vi "Read Permissions.vi"(8 "Error In":errorcluster, 11 "File Info In":refnum<class "File Info.lvclass">) -> (0 "Error Out":errorcluster, 2 "Permissions":T1, 3 "File Info Out":refnum<class "File Info.lvclass">)   [LabVIEW 2021, in "Field_RnD_Services_LIBSSH2_Toolkit.lvlib" / "File Info.lvclass"]
doc: "Gets the POSIX-style filesystem permissions, or mode."
uses:
  220524-VNA RP FLAT.llb/File Info.lvclass
  220524-VNA RP FLAT.llb/Permissions.ctl
  Field_RnD_Services_LIBSSH2_Toolkit/Modes.ctl
  220524-VNA RP FLAT.llb/File Info.lvclass/File Info.ctl
  220524-VNA RP FLAT.llb/Field_RnD_Services_LIBSSH2_Toolkit.lvlib
  220524-VNA RP FLAT.llb/SSH.lvclass
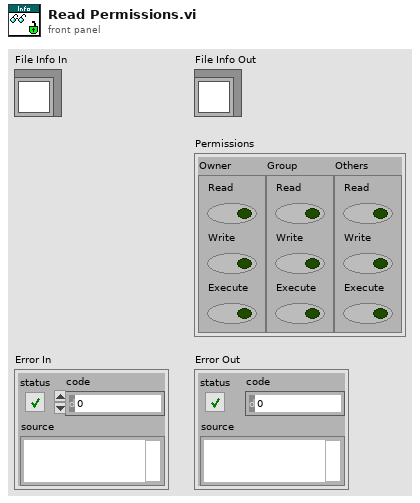
[diagram p1: front panel]
types:
  T1 = typedef "Field_RnD_Services_LIBSSH2_Toolkit.lvlib/Permissions.ctl" = cluster{"Owner":T2, "Group":T2, "Others":T2}
  T2 = typedef "Field_RnD_Services_LIBSSH2_Toolkit.lvlib/Modes.ctl" = cluster{"Read":bool, "Write":bool, "Execute":bool}
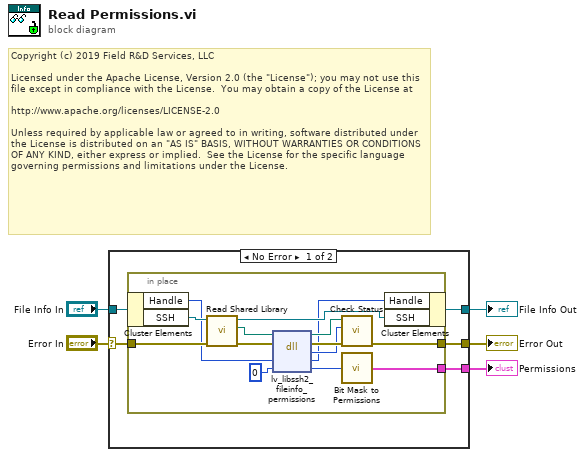
[diagram p0: block diagram]
diagram:
  # "Copyright (c) 2019 Field R&D Services, LLC\n\nLicensed under the Apache License, Version 2.0 (the \"License\"); you may not use this file except in compliance with the License.  You may obtain a copy of the License at\n\nhttp://www.apache.org/licenses/LICENSE-2.0\n\nUnless required by applicable law or agreed to in writing, software distributed under the License is distributed on an \"AS IS\" BASIS, WITHOUT WARRANTIES OR CONDITIONS OF ANY KIND, either express or implied.  See the License for the specific language governing permissions and limitations under the License."
  n1 = case shown="No Error" "Error In" {
    selector: "Error In" -> [w9 w26]
    tunnel: [w7 w26] -> w4
    tunnel: "File Info In" -> [w10 w25]
    tunnel: [w8 w25] -> w2
    tunnel: [w6 _] -> w1
    frame No Error {
      n2 = in-place {
        in-place-border: w9 -> [w17]
        in-place-border: [w14] -> w7
        in-place-border: [w11] -> w6
        n3 = in-place-cluster #1(w10) -> ("Handle"=w16:u64, "SSH"=w21:refnum<class "SSH.lvclass">)
        n4 = call "Read Shared Library.vi"("Error In"=w17, "SSH In"=w21) -> ("Error Out"=w18:errorcluster, "libssh2lv Shared Library"=w19:path, "SSH Out"=w20:refnum<class "SSH.lvclass">)  [unwired: 7 in]
        n5 = dll-call lib="lv-libssh2.*" fn="lv_libssh2_fileinfo_permissions"(path in=w19, error in=w18, "handle"=w16, "permissions"=u32 0 ("flags")) -> (path out=w23:path, error out=w24:errorcluster, "status"=w22:i32, "handle"=w15:u64, "permissions"=w12:u32)  [unwired: 1 in]
        n6 = call "Check Status.vi"("Error In"=w24, "Status"=w22, "libssh2lv Shared Library In"=w23) -> ("Error Out"=w14:errorcluster)  [unwired: 7 in, 1 out]
        n7 = call "Bit Mask to Permissions.vi"("Bit Mask"=w12) -> ("Permissions"=w11:T1)
        n8 = in-place-cluster #1("Handle"=w15, "SSH"=w20) -> (w8:refnum<class "File Info.lvclass">)
      }
    }
    frame Error {
    }
  }
  "Error Out" <- w4
  "File Info Out" <- w2
  "Permissions" <- w1
